vi "st_eval CDF (gamma).vi"(4 "parameters":variant, 5 "x":dbl) -> (2 "f(x)":dbl)   [LabVIEW 2014, in "NI_Gmath.lvlib"]
uses:
  NI_Gmath.lvlib
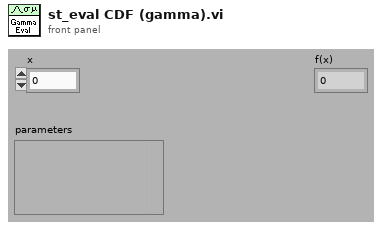
[diagram p1: front panel]
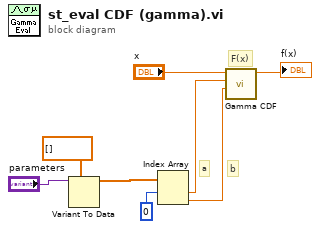
[diagram p0: block diagram]
diagram:
  # "b"
  # "a"
  # "F(x)"
  n1 = Variant To Data(type=dbl[] [], Variant="parameters") -> (data=w6:dbl[])  [unwired: 1 in, 1 out]
  n2 = Index Array(array=w6, index #1=0 ("index")) -> (element #1=w2:dbl, element #2=w1:dbl)  [unwired: 1 in]
  n3 = call "Gamma CDF.vi"("c"=w1, "b"=w2, "x"="x") -> ("cdf(x)"=→"f(x)":dbl)  [unwired: 7 in, 1 out]
